vi "Test_SharedNetworkVariable.vi"(8 "error in (no error)":errorcluster) -> (0 "error out":errorcluster)   [LabVIEW 2013]
uses:
  source/uri/URI.lvclass/URI.ctl
  source/components/path/URI-Component.Path.lvclass/URI-Component.Path.ctl
  source/components/path/URI-Component.Path.lvclass
  source/uri/Read scheme.vi
  source/uri/Read host.vi
  source/uri/Read path.vi
  source/uri/Read path segments.vi
  source/components/path/Get Segments.vi
  <vilib>/addons/_JKI Toolkits/Caraya/classes/Assert/Assert Equal Value_Variant.vi
  source/components/path/Get path (absolute).vi
  <vilib>/addons/_JKI Toolkits/Caraya/classes/Test/Test.lvclass
  <vilib>/addons/_JKI Toolkits/Caraya/classes/Assert/Assert.lvclass
  source/uri/URI.lvclass
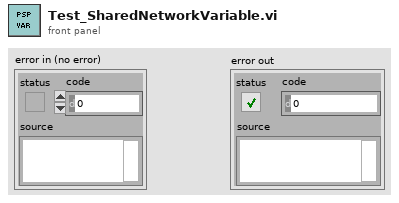
[diagram p1: front panel]
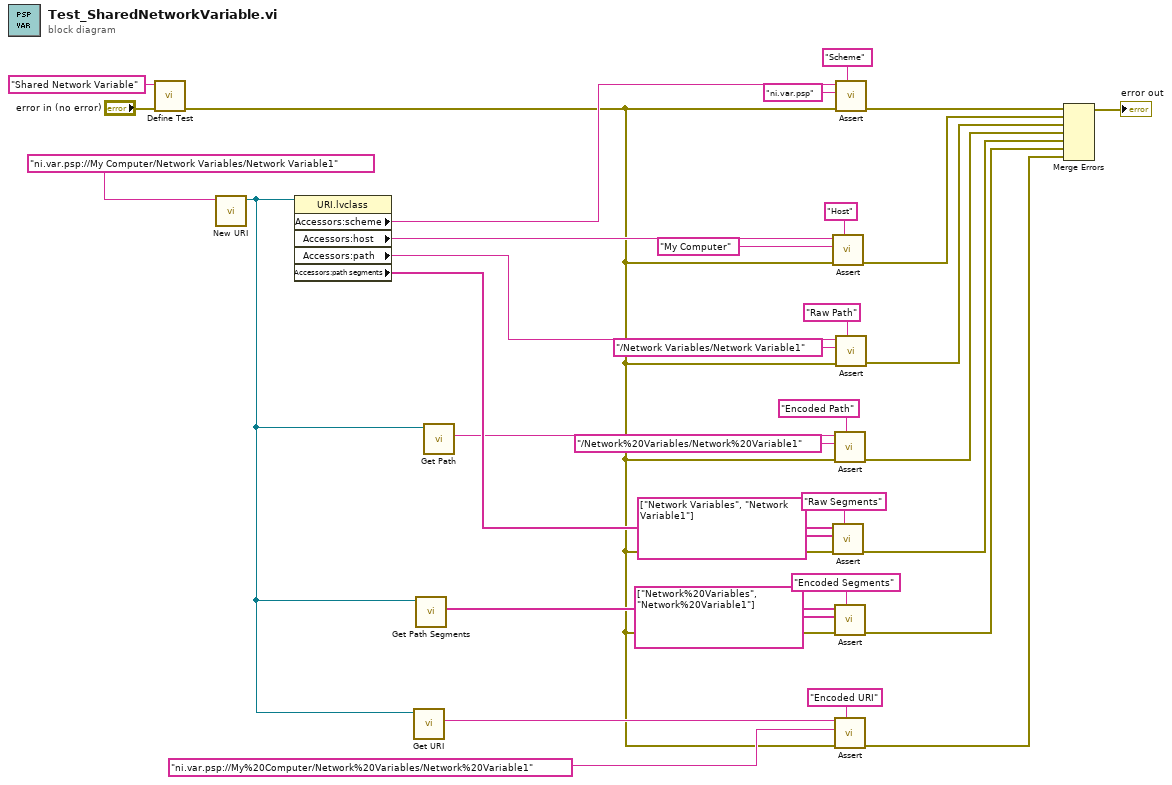
[diagram p0: block diagram]
diagram:
  n1 = call <vilib>:"Define Test.vi"("error in (no error)"="error in (no error)", "Label (VI Title)"="Shared Network Variable") -> ("error out"=w4:errorcluster)  [unwired: 9 in]
  n2 = call "New URI.vi"("URI"="ni.var.psp://My Computer/Network Variables/Network Variable1") -> ("URI"=w3:refnum<class "URI.lvclass">)  [unwired: 9 in, 1 out]
  n3 = property on="Property Node" class="URI.lvclass"(reference=w3) -> ("Accessors:scheme"=w29:string, "Accessors:host"=w18:string, "Accessors:path"=w17:string, "Accessors:path segments"=w9:string[])  [unwired: 1 in, 2 out]
  n4 = call "Get URI.vi"("URI in"=w3) -> ("URI String"=w14:string)  [unwired: 8 in, 2 out]
  n5 = call "Get Path Segments.vi"("URI in"=w3) -> ("Segments"=w7:string[])  [unwired: 8 in, 2 out]
  n6 = call "Get Path.vi"("URI in"=w3) -> ("path"=w2:string)  [unwired: 8 in, 2 out]
  n7 = call-poly <vilib>:"Assert.vi"("Label"="Host" ("URI"), "error in (no error)"=w4, "Y"="My Computer" ("URI"), "X"=w18) -> ("error out"=w25:errorcluster)  [unwired: 7 in]
  n8 = call-poly <vilib>:"Assert.vi"("Label"="Raw Segments" ("URI"), "error in (no error)"=w4, "Y"=string[] ["Network Variables", "Network Variable1"] ("Segments"), "X"=w9) -> ("error out"=w8:errorcluster)  [unwired: 7 in]
  n9 = call-poly <vilib>:"Assert.vi"("Label"="Encoded Path" ("URI"), "error in (no error)"=w4, "Y"="/Network%20Variables/Network%20Variable1" ("URI"), "X"=w2) -> ("error out"=w1:errorcluster)  [unwired: 7 in]
  n10 = call-poly <vilib>:"Assert.vi"("Label"="Encoded Segments" ("URI"), "error in (no error)"=w4, "Y"=string[] ["Network%20Variables", "Network%20Variable1"] ("Segments"), "X"=w7) -> ("error out"=w19:errorcluster)  [unwired: 7 in]
  n11 = call-poly <vilib>:"Assert.vi"("Label"="Encoded URI" ("URI"), "error in (no error)"=w4, "Y"="ni.var.psp://My%20Computer/Network%20Variables/Network%20Variable1" ("URI"), "X"=w14) -> ("error out"=w12:errorcluster)  [unwired: 7 in]
  n12 = call-poly <vilib>:"Assert.vi"("Label"="Scheme" ("URI"), "error in (no error)"=w4, "Y"="ni.var.psp" ("URI"), "X"=w29) -> ("error out"=w26:errorcluster)  [unwired: 7 in]
  n13 = call-poly <vilib>:"Assert.vi"("Label"="Raw Path" ("URI"), "error in (no error)"=w4, "Y"="/Network Variables/Network Variable1" ("URI"), "X"=w17) -> ("error out"=w22:errorcluster)  [unwired: 7 in]
  n14 = Merge Errors(w26, w25, w22, w1, w8, w19, w12) -> (→"error out":errorcluster)
